vi "StateSpaceUtil_MakeCostMatrix.vi"(7 "States":i32, 11 "Costs":T1) -> (3 "Costs Matrix":T1)   [LabVIEW 2019, in "Trajectory_Library.lvlib"]
doc: "Creates a new LINEAR SYSTEM data cluster with the specified values. \n\n\nInputs: \n - XXX -- XXX.\n\nOutputs:\n - XXX -- XXX."
uses:
  Trajectory_Library.lvlib
  <vilib>/Analysis/Matrix/Datatypes/RealMatrix.ctl
  <vilib>/Analysis/Matrix/NI_Matrix.lvlib
panel:
  # "<States,States>"
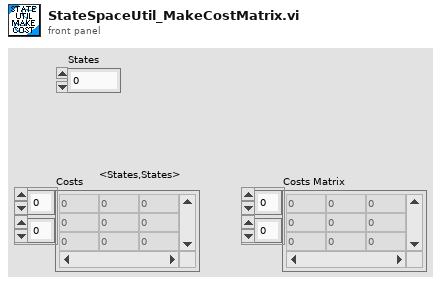
[diagram p1: front panel]
types:
  T1 = typedef "NI_Matrix.lvlib/RealMatrix.ctl" = dbl[][]
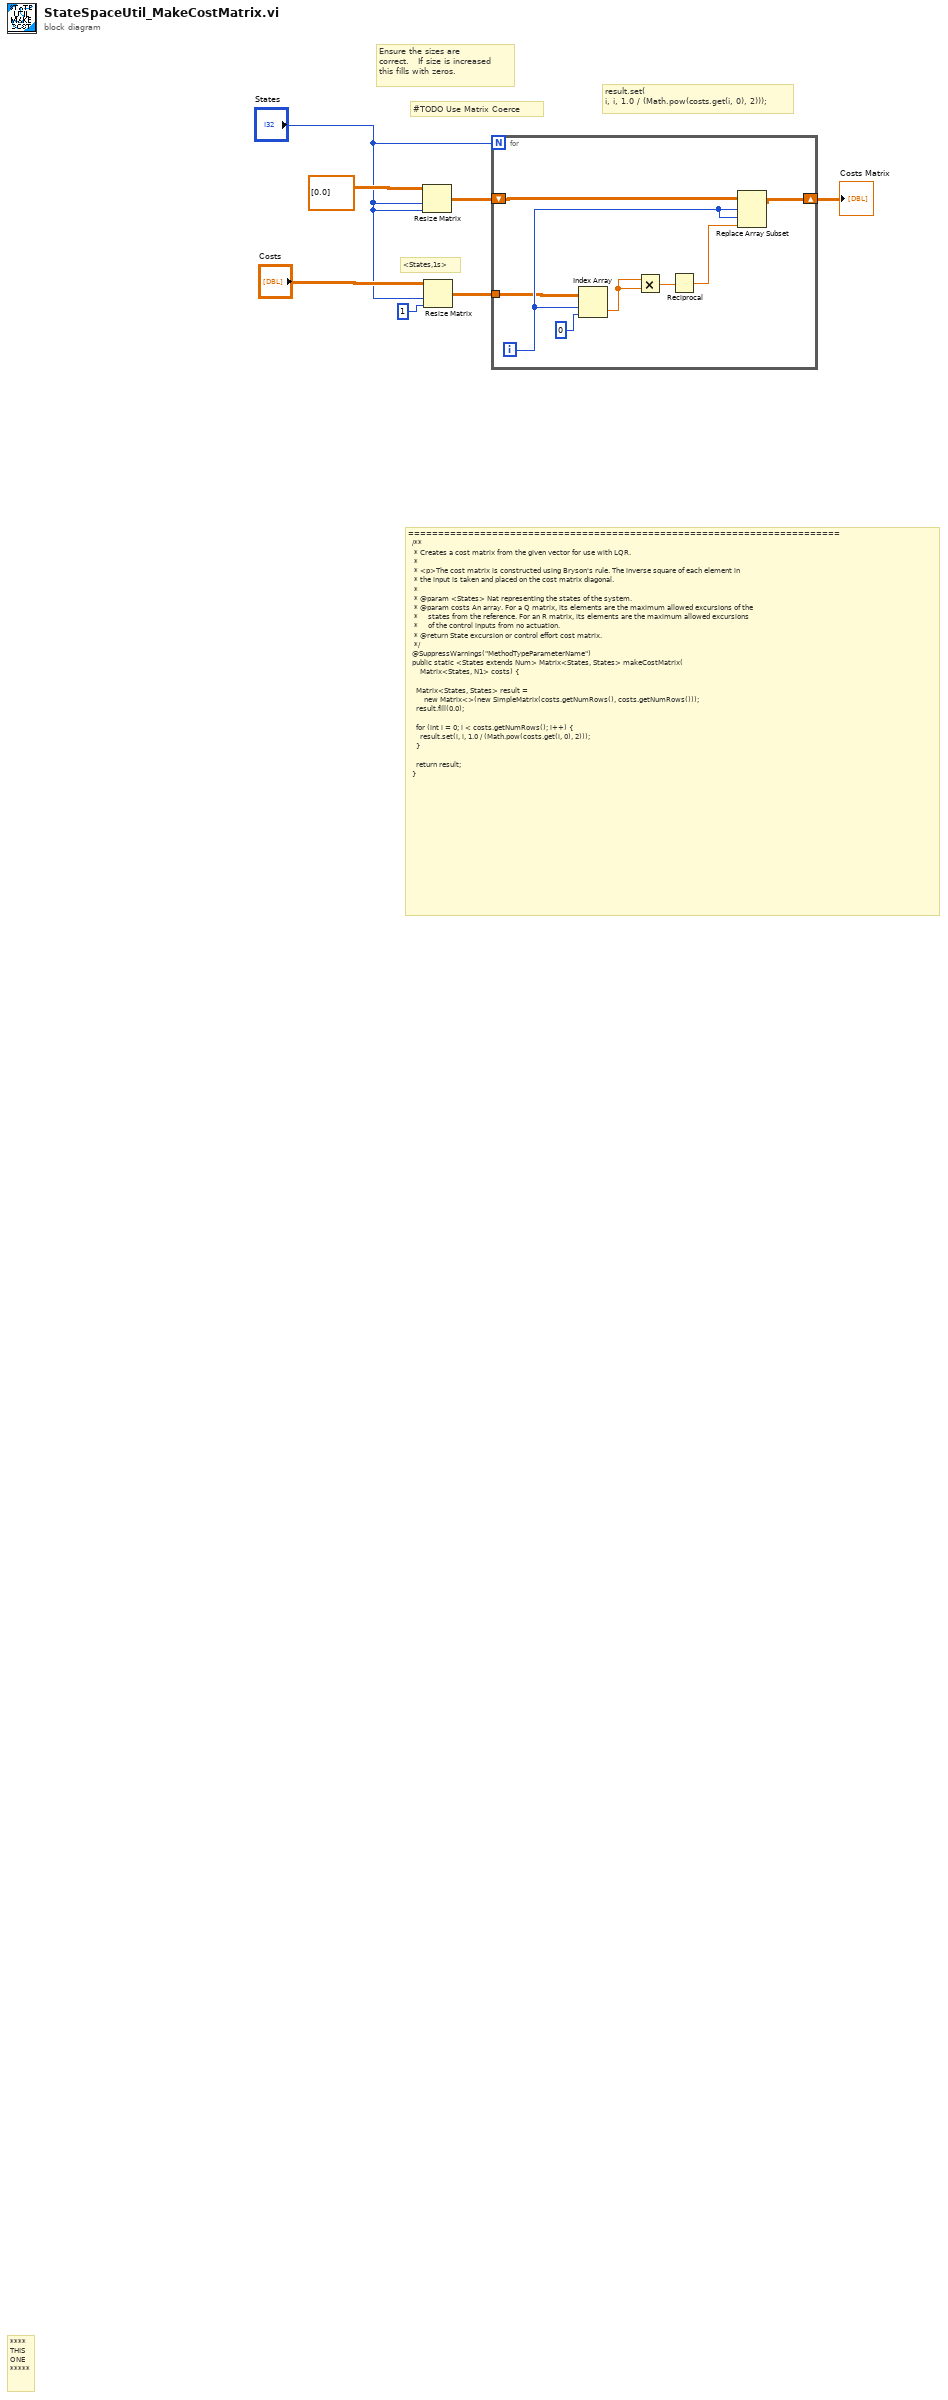
[diagram p0: block diagram]
diagram:
  # "#TODO Use Matrix Coerce"
  # "result.set(\ni, i, 1.0 / (Math.pow(costs.get(i, 0), 2)));"
  # "========================================================================\n  /**\n   * Creates a cost matrix from the given vector for use with LQR.\n   *\n   * <p>The cost matrix is constructed using Bryson's rule. The inverse square of each element in\n   * the input is taken and placed on the cost matrix diagonal.\n   *\n   * @param <States> Nat representing the states of the system.\n   * @param costs An array. For a Q matrix, its elements are the maximum allowed excursions of the\n   *     states from the reference. For an R matrix, its elements are the maximum allowed excursions\n   *     of the control inputs from no actuation.\n   * @return State excursion or control effort cost matrix.\n   */\n  @SuppressWarnings(\"MethodTypeParameterName\")\n  public static <States extends Num> Matrix<States, States> makeCostMatrix(\n      Matrix<States, N1> costs) {\n\n    Matrix<States, States> result =\n        new Matrix<>(new SimpleMatrix(costs.getNumRows(), costs.getNumRows()));\n    result.fill(0.0);\n\n    for (int i = 0; i < costs.getNumRows(); i++) {\n      result.set(i, i, 1.0 / (Math.pow(costs.get(i, 0), 2)));\n    }\n\n    return result;\n  }"
  # "<States,1s>"
  # "Ensure the sizes are\ncorrect.   If size is increased \nthis fills with zeros."
  # "****\nTHIS\nONE\n*****"
  n1 = Resize Matrix(1:"States", 2:"States", 4:T1 [[0.0]] ("Costs")) -> (0:w4:T1)
  n2 = Resize Matrix(1:1 ("number of columns"), 2:"States", 4:"Costs") -> (0:w3:T1)
  n3 = for {
    N: "States" -> [_]
    tunnel: w3 -> [w11]
    shift-right: [w15] -> w1
    shift-left: w4 -> [w14]
    i -> [w13]
    n4 = Index Array(array=w11, index (row)=w13, index (col)=0) -> (element=w10:dbl)
    n5 = Multiply(x=w10, y=w10) -> (x*y=w9:dbl)
    n6 = Reciprocal(x=w9) -> (1/x=w8:dbl)
    n7 = Replace Array Subset(array=w14, new element=w8, index (row)=w13, index (col)=w13) -> (w15:T1)
  }
  "Costs Matrix" <- w1
